vi "Query Fault Table.vi"(0 "GEA2 Reference In":refnum<k24>, 2 "Standalone?":bool, 5 "GEA Inputs":T1={"Source"=228, "Destination"=35} {"Destination" format="%.0x"; "Source" format="%.0x"}, 7 "Fault ID":u16, 11 "Error In":errorcluster) -> (4 "GEA2 Reference Out":refnum<k24>, 6 "Fault Status":string, 15 "Error Out":errorcluster)   [LabVIEW 2016, in "Centauro.lvlib"]
uses:
  Projects/Centauro.lvlib
  Common/LabVIEW GEA2 Toolkit/LabVIEW_GEA2_Toolkit.lvlibp/type defs/Source_Destination.ctl
  Q:/Common/DLLs/GEA3/GeaCommunication.dll
  Common/DLLs/GEA3/GeaCommunication.dll
  Common/LabVIEW GEA2 Toolkit/LabVIEW_GEA2_Toolkit.lvlibp/type defs/ERD Read Data In.ctl
  Common/LabVIEW GEA2 Toolkit/LabVIEW_GEA2_Toolkit.lvlibp/type defs/Data Type.ctl
  Common/LabVIEW GEA2 Toolkit/LabVIEW_GEA2_Toolkit.lvlibp
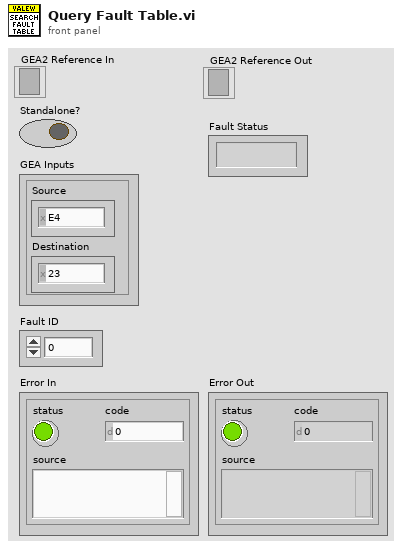
[diagram p1: front panel]
types:
  T1 = typedef "LabVIEW_GEA2_Toolkit.lvlibp/Source_Destination.ctl" = cluster{"Source":u8, "Destination":u8}
  T2 = typedef "LabVIEW_GEA2_Toolkit.lvlibp/ERD Read Data In.ctl" = cluster{"ERD Number":u16, "Data Type":T3}
  T3 = typedef "LabVIEW_GEA2_Toolkit.lvlibp/Data Type.ctl" = enum16{"string", "boolean", "uint8_t", "uint16_t", "uint32_t", "uint64_t", "int8_t", "int16_t", "int32_t", "int64_t"}
  T4 = typedef "LabVIEW_GEA2_Toolkit.lvlibp/ERD Read Data Out.ctl" = cluster{"ERD Number":u16, "Data":string}
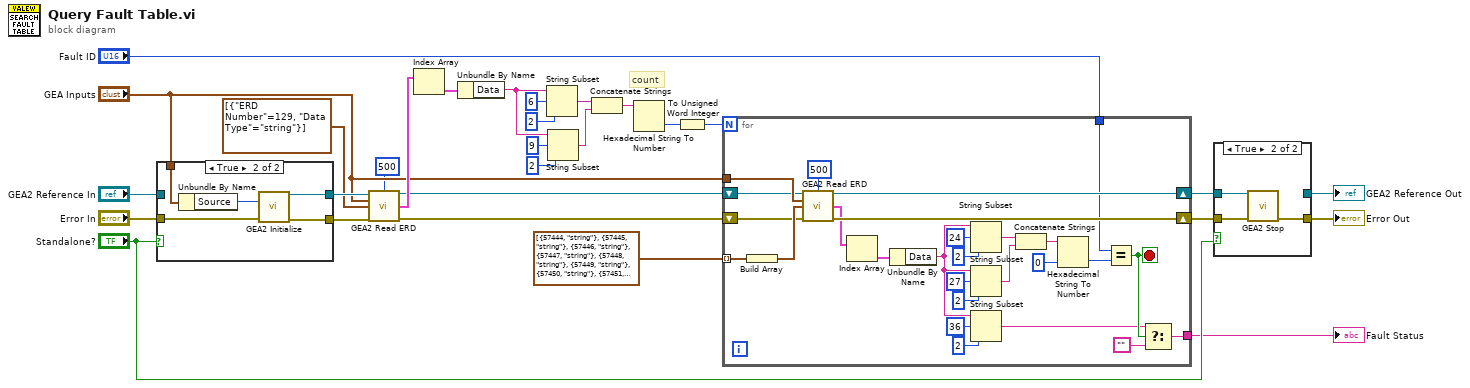
[diagram p0: block diagram]
diagram:
  # "count"
  n1 = case shown="True" "Standalone?" {
    tunnel: [w30 w36] -> w19
    tunnel: [w31 w35] -> w18
    tunnel: "GEA Inputs" -> [_ w34]
    tunnel: "Error In" -> [w31 w32]
    tunnel: "GEA2 Reference In" -> [w30 _]
    frame False {
    }
    frame True {
      n2 = Unbundle By Name(w34) -> ("Source"=w33:u8)
      n3 = call "GEA2 Initialize.vi"("Source Address"=w33, "error in"=w32) -> ("GEA2 Reference Out"=w36:refnum<k24>, "error out"=w35:errorcluster)  [unwired: 11 in, 1 out]
    }
  }
  n4 = call "GEA2 Read ERD.vi"("GEA2 Reference In"=w19, "Read Timeout (ms)"=u32 500, "GEA Inputs"="GEA Inputs", "Read ERD List"=T2[] [{"ERD Number"=129, "Data Type"=enum."string"}], "Error In"=w18) -> ("GEA2 Reference Out"=w14:refnum<k24>, "ERD Data Out"=w20:T4[], "Error Out"=w11:errorcluster)  [unwired: 7 in, 1 out]
  n5 = Index Array(array=w20) -> (element=w21:T4)  [unwired: 1 in]
  n6 = Unbundle By Name(w21) -> ("Data"=w26:string)
  n7 = String Subset(string=w26, offset (0)=6, length (rest)=2 ("length (rest)")) -> (substring=w25:string)
  n8 = String Subset(string=w26, offset (0)=9, length (rest)=2 ("length (rest)")) -> (substring=w24:string)
  n9 = Concatenate Strings(w25, w24) -> (w23:string)
  n10 = Hexadecimal String To Number(string=w23) -> (number=w22:u32)  [unwired: 2 in, 1 out]
  n11 = To Unsigned Word Integer(number=w22) -> (unsigned 16bit integer=w16:u16)
  n12 = for {
    N: w16 -> [_]
    shift-right: [w57] -> w12
    shift-left: w11 -> [w60]
    shift-right: [w58] -> w13
    shift-left: w14 -> [w59]
    tunnel: T2[] [{"ERD Number"=57444, "Data Type"=enum."string"}, {"ERD Number"=57445, "Data Type"=enum."string"}, {"ERD Number"=57446, "Data Type"=enum."string"}, {"ERD Number"=57447, "Data Type"=enum."string"}, {"ERD Number"=57448, "Data Type"=enum."string"}, {"ERD Number"=57449, "Data Type"=enum."string"}, {"ERD Number"=57450, "Data Type"=enum."string"}, {"ERD Number"=57451, "Data Type"=enum."string"}, {"ERD Number"=57452, "Data Type"=enum."string"}, {"ERD Number"=57453, "Data Type"=enum."string"}] ("Read ERD List") -> [w63] mode=indexing
    tunnel: "GEA Inputs" -> [w61]
    tunnel: "Fault ID" -> [w45]
    tunnel: [w39] -> w5
    stop <- w41 stop-if-true
    n13 = Build Array(w63) -> (w62:T2[])
    n14 = call "GEA2 Read ERD.vi"("GEA2 Reference In"=w59, "Read Timeout (ms)"=u32 500, "GEA Inputs"=w61, "Read ERD List"=w62, "Error In"=w60) -> ("GEA2 Reference Out"=w58:refnum<k24>, "ERD Data Out"=w56:T4[], "Error Out"=w57:errorcluster)  [unwired: 7 in, 1 out]
    n15 = Index Array(array=w56) -> (element=w55:T4)  [unwired: 1 in]
    n16 = Unbundle By Name(w55) -> ("Data"=w42:string)
    n17 = String Subset(string=w42, offset (0)=24, length (rest)=2 ("length (rest)")) -> (substring=w52:string)
    n18 = String Subset(string=w42, offset (0)=27, length (rest)=2 ("length (rest)")) -> (substring=w51:string)
    n19 = String Subset(string=w42, offset (0)=36, length (rest)=2 ("length (rest)")) -> (substring=w40:string)
    n20 = Concatenate Strings(w52, w51) -> (w50:string)
    n21 = Hexadecimal String To Number(string=w50, default (0uL)=u16 0 ("offset (0)")) -> (number=w47:u16)  [unwired: 1 in, 1 out]
    n22 = Equal?(x=w45, y=w47) -> (x = y?=w41:bool)
    n23 = Select(t=w40, s=w41, f="") -> (s? t:f=w39:string)
  }
  "Fault Status" <- w5
  n24 = case shown="True" "Standalone?" {
    tunnel: w13 -> [w64 w68]
    tunnel: w12 -> [w65 w67]
    tunnel: [w65 w66] -> w2
    tunnel: [w64 _] -> w4
    frame False {
    }
    frame True {
      n25 = call "GEA2 Stop.vi"("GEA2 Reference In"=w68, "Error In"=w67) -> ("Error Out"=w66:errorcluster)  [unwired: 13 in]
    }
  }
  "GEA2 Reference Out" <- w4
  "Error Out" <- w2
